vi "sub_measure_total-length.vi"(11 "TM graph":cluster{"lat":dbl, "long":dbl}[](array[cluster])) -> (3 "totol length":dbl)   [LabVIEW 2019]
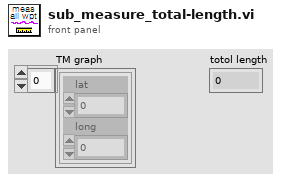
[diagram p1: front panel]
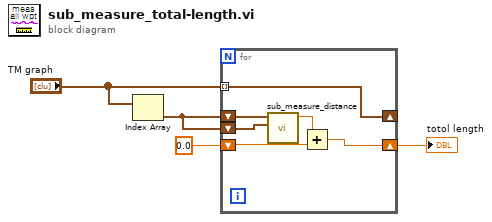
[diagram p0: block diagram]
diagram:
  n1 = Index Array(array="TM graph") -> (element=w3:cluster{"lat":dbl, "long":dbl})  [unwired: 1 in]
  n2 = for {
    tunnel: "TM graph" -> [w10] mode=indexing
    shift-right: [w10] -> _
    shift-left: w3 -> [w9]
    shift-left: w3 -> [w8]
    shift-right: [w5] -> w1
    shift-left: 0.0 -> [w7]
    n3 = call "sub_measure_distance.vi"("pt 2"=w8, "pt 1"=w9) -> ("distance"=w6:dbl)  [unwired: 9 in]
    n4 = Add(x=w6, y=w7) -> (x+y=w5:dbl)
  }
  "totol length" <- w1
